vi "V7310.Main-Start.vi"(8 "error in":errorcluster, 9 "Wait (T)":bool=TRUE, 10 "Job":T1) -> (0 "error out":errorcluster, 2 "Aborted":bool)   [LabVIEW 2015]
uses:
  LowLevel/V7310.Job.Data.ctl
  LowLevel/V7310.Job.Sets.ctl
  tools/EventLog/EventLog.EventSource.ctl
  tools/Translator/Translator.Message.ctl
  V7310.Action.ctl
  V7310.Data.Status.State.ctl
  LowLevel/V7310.LaserStatus.ctl
  tools/EventLog/EventLog.CreateError(array).vi
  tools/Translator/Translator.Translate.Status (NoError).vi
  tools/Translator/Translator.FormatMessage.vi
  LowLevel/V7310.Global.vi
  tools/Translator/Translator.Global.vi
  tools/ErrorHandling/ErrorHandling.Create.vi
  tools/EventLog/EventLog.CreateError(single).vi
panel:
  out "delays":u32[](array[numeric])
  out "idx":i32
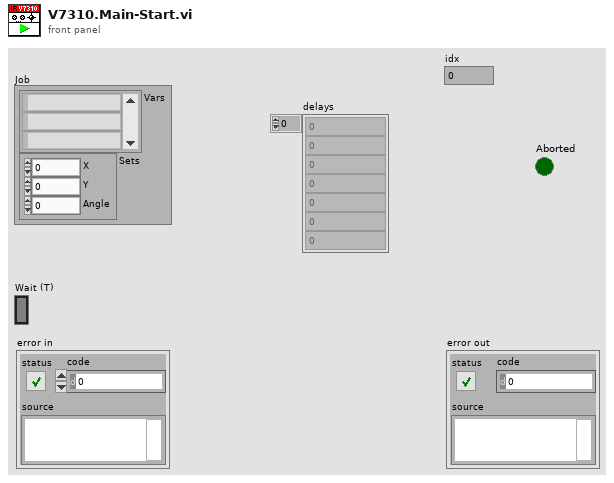
[diagram p1: front panel]
types:
  T1 = typedef "V7310.Job.Data.ctl" = cluster{"Vars":string[], "Sets":T2}
  T2 = typedef "V7310.Job.Sets.ctl" = cluster{"X":dbl, "Y":dbl, "Angle":dbl}
  T3 = typedef "EventLog.EventSource.ctl" = enum16{"All", "Gui", "Ref", "File", "Arch", "Seq", "CPX", "Proda", "Laser", "Scan.P", "Scan.O"}
  T4 = typedef "Translator.Message.ctl" = enum16{"-", "Event confirmed", "Log out", "Log in", "Shutdown", "Cancel", "Start", "Begin time", "End time", "Duration", "Service Mode", "Ignore Results", "On", "Off", "OK", "NOK", "NOK %s", "Home", "Work", "Close", "Open", "In progress...", "Missing", "Empty", "Hardware failure", "Initial", "Out of range", "Error %d >> %s", "Error %d >> %s >> %s", "Msg %d >> %s", "Laser msg %d %s", "Laser cmd error %s %d", "Laser cmd failed %s", "Laser cmd warning %s", "Laser disconnected", "Laser status %s", "Laser already started", "Laser job unkonwn %s", "Laser job missing %s", "Laser job select failure %s", "Unable to start laser printing (%s)", "Unable to stop laser printing (%s)", "Laser marking aborted", "Laser marking timeout", "Unable to reset Laser Interlock (%s)", "Unable to trigger Laser. Laser not ready (%s)", "Laser job '%s' coordinates not configured", "Starting %s", "Quitting %s", "Configured", "Initializing", "Quitting", "Loading", "Running", "Stopped", "Summary", "Laser", "Do you want to continue?", "Press confirm button", "Station is not based. Do you want to exit?", "Station requires changeover. Do you want to run the test?", "Test options are not set as default. Do you want to continue?", "Product not detected. Do you want to continue?", "Product scan failed. Do you want to continue?", "Calibration", "Log out?", "System", "All", "IDLE", "Translating...%s", "Not found", "Alarm %s", "Run", "Skip", "Abort", "Repeat", "Please wait...", "Database disconnected", "Database disconnected - changeover disabled!", "Login to database successful", "Login to database failed: %d; %s", "Unable to check the product status of reference %d - database disconnected", "Unable to set the product status of reference %d - database disconnected", "Variant file backup %s", "Read steps (%s)", "Result", "Station armed!", "Station requires changeover!", "Select reference number...", "EMERGENCY BUTTON - press Control button", "EMERGENCY DOOR - press Control button", "Resetting Emergency...", "Unable to reset safety circuit - Emergency Button pressed", "Unable to reset safety circuit - Emergency Side Door open", "Station not based", "Station based", "Station not empty", "Station basing...", "No order", "Press Start to begin new order", "Scanning new order", "Order NOK. Correct or scan again", "Order OK. Press Accept", "Order ready", "Revolver incorrect", "Fork incorrect", "Revolver missing", "Revolver empty", "Container missing", "Offline results", "Door open", "Close the front door", "Press start button", "Done. Open the front door", "Running...", "Running...%.1f %%", "Pause", "Pause. NOK container missing", "Pause. OK container missing", "Pause. Revolver empty", "Pause. Revolver missing", "Pause. Revolver incorrect", "Pause. Fork missing", "Pause. Fork incorrect", "Pause. Too many failures", "Pause. One slot is not working", "Pause. Unable to move product to slot", "Pause. Unable to move back product pusher", "Pause. Unable to lift product", "Pause. Unable to move back product lifter", "Pause. Unable to move product arm to Work", "Pause. Unable to move product arm to NOK", "Pause. Unable to move product arm to OK", "Pause. Unable to unsuck the NOK product", "Pause. Unable to drop the NOK product", "Pause. Product OK missing", "Pause. Unable to unsuck the OK product", "Pause. Unable to drop the OK product", "Stopping...", "File '%s' is missing", "File '%s' is broken", "File '%s' is running", "Log file started (%s)", "Log file ended (%s)", "Log file ignored (%s)", "Log file exported (%s)", "Log file export failed (%s)", "Wrong serial number in log file", "Wrong reference number in log file", "Test steps are missing", "%s = %.3f", "Process param '%s' not found in DB", "Process param '%s' wrong order", "Process param '%s' value %.3f out of limits (%.3f; %.3f)", "Step%d param '%s' not found in DB", "Step%d param '%s' wrong order", "Step%d param '%s' value %.3f out of limits (%.3f; %.3f)", "Step%d EV '%s' not found in DB", "Step%d EV '%s' wrong order", "\"%s\" not found in DB", "\"%s\" wrong order", "\"%s\" value %.3f out of limits (%.3f; %.3f)", "\"%s\" not found in software", "Process init (%s)", "Process started", "Process restarted", "Process run", "Process done", "Process aborted", "Process aborted at work", "Process aborted at home", "Process error", "Process error at home", "Process error at work", "Process close", "Select plate from the order to process", "Do you want to start the process?", "Do you want to repeat the process?", "There is unfinished order. Do you want to put the new order?", "Product %s %d OK", "Product %s %d NOK", "Unable to unload the slot %s. Product missing in the slot", "Unable to unload the slot %s. Product already in the arm", "Unable to accept the product as OK. Product missing in slot %s", "Unable to accept the product as OK. Product could not drop into the container at slot %s", "Unable to accept the product as NOK. Product could not drop into the container at slot %s", "Scan failed. Error %s", "Scan failed. Scanner disconnected", "Scan failed. Wrong Wabco number %d, limit (%d,%d)", "Scan failed. Wrong serial number %d, limit (%d,%d)", "Scan failed. Wrong date %d, limit (%d,%d)", "Scan failed. Wrong product wabco number %d (expected %d)", "Scan failed. Wrong product serial number %d (expected > 0)", "Scan OK %s", "Scan failed. Unable to determine table position (%s)", "Scan failed. Timeout", "Tune failed. Scanner disconnected", "Tune failed. Timeout", "%s = %d", "%s = %d->%d", "Unable to set %s = %.2f - Air Pressure Inside off", "Unable to set digital output '%s' = %d", "Unable to activate air pressure inside - timeout", "Unable to activate air pressure inside - aborted", "Unable to switch on Air Main Valve - Air Pressure Inlet off", "Unable to switch on Air Main Valve - Door open", "Unable to switch off Air Main Valve - timeout", "Unable to switch off Air Main Valve - aborted", "Unable to rotate Table - timeout", "Unable to rotate Table - aborted", "Unable to rotate Table - Product Move not in Home position", "Unable to rotate Table - Air Pressure Inside off", "Unable to rotate Table - Product Lift A not in Home position", "Unable to rotate Table - Product Lift B not in Home position", "Unable to rotate Table - unlock before movement timeout", "Unable to rotate Table - lock after movement timeout", "Unable to move Table Lock to %s position - timeout", "Unable to move Table Lock to %s position - aborted", "Unable to move Table Lock to %s position - Air Pressure Inside off", "Unable to move Table Lock to %s position - Table not in position", "Unable to move Product Lift A to %s position - timeout", "Unable to move Product Lift B to %s position - timeout", "Unable to move Product Lift A to %s position - aborted", "Unable to move Product Lift B to %s position - aborted", "Unable to move Product Lift A to %s position - Air Pressure Inside off", "Unable to move Product Lift B to %s position - Air Pressure Inside off", "Unable to move Product Lift A to %s position - Table not locked", "Unable to move Product Lift B to %s position - Table not locked", "Unable to move Product Lift A to %s position - Product Arm not in Work position", "Unable to move Product Lift B to %s position - Product Arm not in Work position", "Unable to set Product Suction Gripper %s to %s - timeout", "Unable to set Product Suction Gripper %s to %s - aborted", "Unable to set Product Suction Gripper %s to %s - Air Pressure Inside off", "Unable to set Product Suction Gripper %s to %s - Table slot unkown", "Unable to move Product Arm to %s position - timeout", "Unable to move Product Arm to %s position - aborted", "Unable to move Product Arm to %s position - Air Pressure Inside off", "Unable to move Product Arm to %s position - Product Lift A not in Home position", "Unable to move Product Arm to %s position - Product Lift B not in Home position", "Unable to move Product to %s position - timeout", "Unable to move Product to %s position - aborted", "Unable to move Product to %s position - Air Pressure Inside off", "Unable to move Product to %s position - Table not in position"}
  T5 = typedef "V7310.Action.ctl" = enum32{"idle", "constructor", "destructor", "--- V7310 ---", "Init", "Select", "Start", "Stop"}
  T6 = typedef "V7310.Data.Status.State.ctl" = enum16{"First", "Init", "Msg", "Error", "Abort", "Idle", "Run"}
  T7 = typedef "V7310.LaserStatus.ctl" = enum16{"-", "FatalError", "Initialize", "KeySwitchOpen", "TimeoutInterlock", "InterlockOpen", "StartUp", "ShutterlockOpen", "Standby", "Ready", "PrepareForMarking", "WaitForTrigger", "Marking"}
  T8 = typedef "V7310.Data.Status.ctl" = cluster{"State":T6, "LaserStatus":T7, "LaserStatusRaw":string, "Ref":refnum<k5>, "RTC TS":timestamp, "Conn TS":timestamp, "Msg":T9[], "JobInUse":string, "Jobs":string[], "Vars":T10[]}
  T9 = typedef "V7310.Message.Data.ctl" = cluster{"ID":i32, "Msg":string}
  T10 = typedef "V7310.Job.Variable.ctl" = cluster{"Name":string, "Value":string}
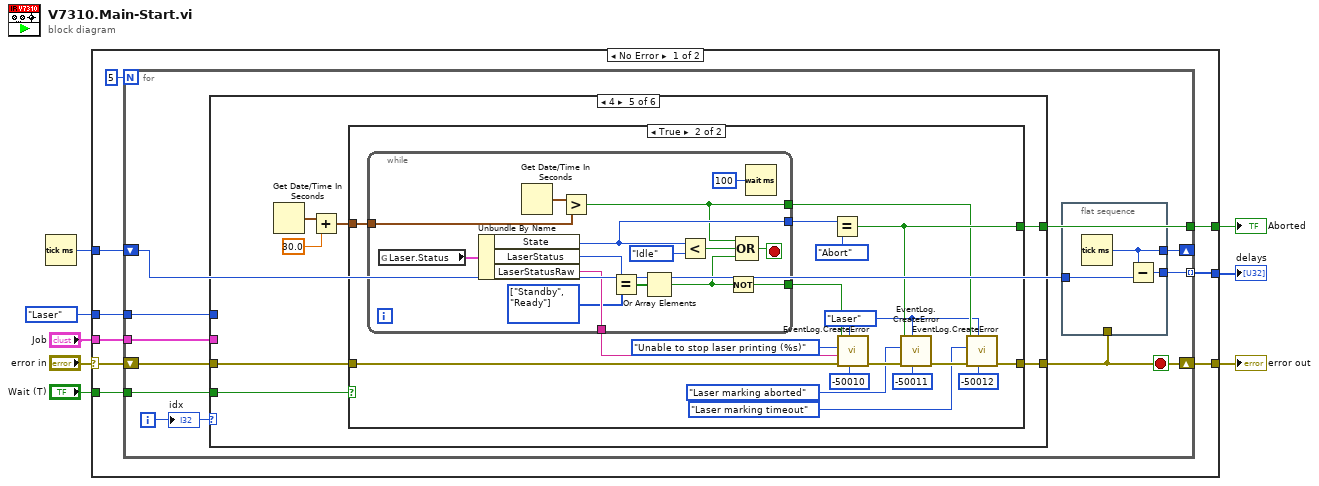
[diagram p0: block diagram]
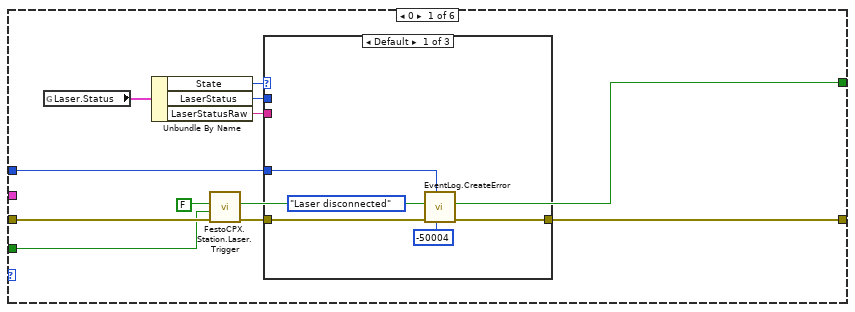
[diagram p2: hidden frame]
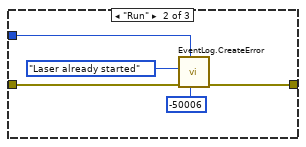
[diagram p3: hidden frame]
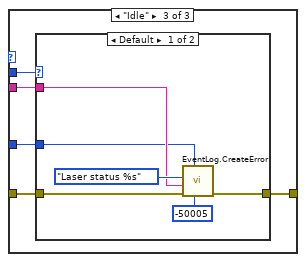
[diagram p4: hidden frame]
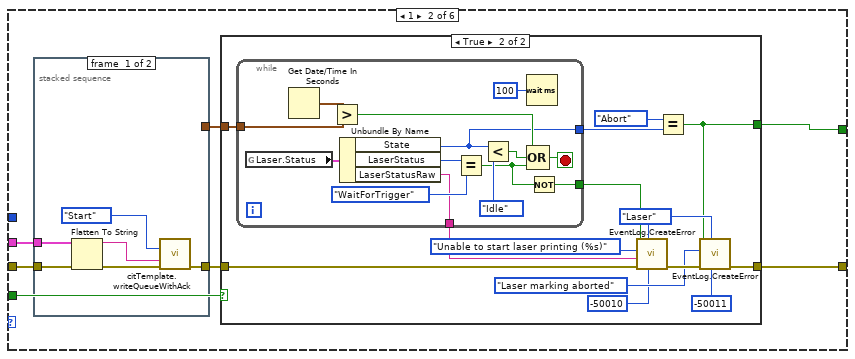
[diagram p6: hidden frame]
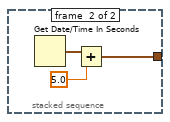
[diagram p7: hidden frame]
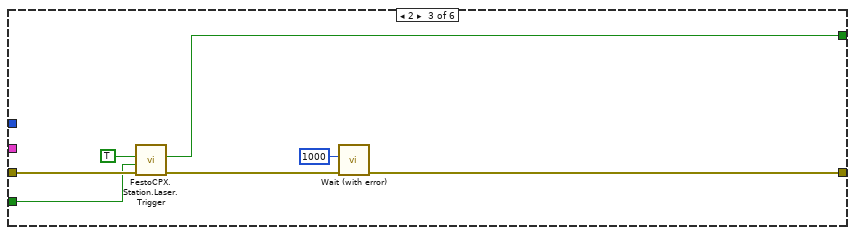
[diagram p9: hidden frame]
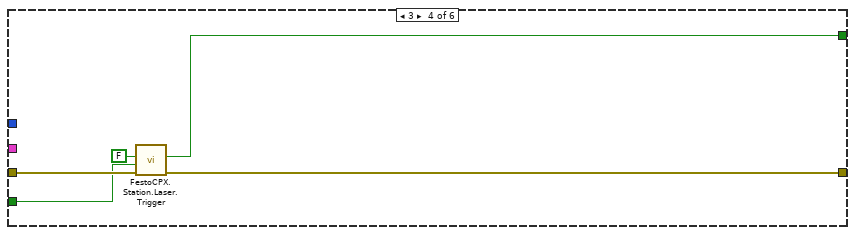
[diagram p10: hidden frame]
diagram:
  n1 = Tick Count (ms)() -> (millisecond timer value=w2:u32)
  n2 = case shown="No Error" "error in" {
    selector: "error in" -> [w15 w163]
    tunnel: [w16 w163] -> w7
    tunnel: "Job" -> [w17 _]
    tunnel: "Wait (T)" -> [w14 _]
    tunnel: [w11 _] -> w4
    tunnel: EventLog.EventSource."Laser" ("Source (All)") -> [w13 _]
    tunnel: w2 -> [w10 _]
    tunnel: [w9 _] -> w1
    frame No Error {
      n3 = for {
        N: 5 -> [_]
        tunnel: w17 -> [w27]
        shift-right: [w21] -> w16
        shift-left: w15 -> [w26]
        tunnel: w14 -> [w25]
        tunnel: w13 -> [w23]
        tunnel: [w22] -> w11
        shift-right: [w20] -> _
        shift-left: w10 -> [w19]
        tunnel: [w18] -> w9 mode=indexing
        i -> [w24]
        stop <- w21 stop-if-true
        n4 = case shown="4" w24 {
          tunnel: w27 -> [_ w70 _ _ _ _]
          tunnel: [w41 w65 w110 w118 w125 w162] -> w21
          tunnel: w26 -> [w37 w69 w114 w119 w121 w162]
          tunnel: w25 -> [w32 w68 w112 w117 w127 _]
          tunnel: w23 -> [w34 _ _ _ _ _]
          tunnel: [w31 w64 w111 w116 w124 _] -> w22
          frame 0 {
            n5 = global read "V7310.Global.vi" "Laser.Status"() -> (w33:T8)
            n6 = Unbundle By Name(w33) -> ("State"=w40:T6, "LaserStatus"=w39:T7, "LaserStatusRaw"=w38:string)
            n7 = call "FestoCPX.Station.Laser.Trigger.vi"("error in"=w37, "Wait (T)"=w32, "Trigger"=FALSE) -> ("error out"=w36:errorcluster, "Aborted"=w31:bool)  [unwired: 7 in]
            n8 = case shown="Default" w40 {
              tunnel: w36 -> [w44 w50 w56]
              tunnel: [w43 w49 w55] -> w41
              tunnel: w39 -> [_ _ w54]
              tunnel: w38 -> [_ _ w53]
              tunnel: w34 -> [w42 w47 w52]
              frame Default {
                n9 = call-poly "EventLog.CreateError.vi"("Code (-1)"=-50004 ("error code (0)"), "Source (All)"=w42, "error in"=w44, "msg"=Translator.Message."Laser disconnected") -> ("error out"=w43:errorcluster)  [unwired: 6 in, 1 out]
              }
              frame "Run" {
                n10 = call-poly "EventLog.CreateError.vi"("Code (-1)"=-50006 ("error code (0)"), "Source (All)"=w47, "error in"=w50, "msg"=Translator.Message."Laser already started") -> ("error out"=w49:errorcluster)  [unwired: 6 in, 1 out]
              }
              frame "Idle" {
                n11 = case shown="Default" w54 {
                  tunnel: w56 -> [w60 w63]
                  tunnel: [w59 w63] -> w55
                  tunnel: w53 -> [w58 _]
                  tunnel: w52 -> [w57 _]
                  frame Default {
                    n12 = call-poly "EventLog.CreateError.vi"("Code (-1)"=-50005 ("error code (0)"), "Source (All)"=w57, "error in"=w60, "arg"=w58, "msg"=Translator.Message."Laser status %s") -> ("error out"=w59:errorcluster)  [unwired: 6 in]
                  }
                  frame "Standby", "Ready" {
                  }
                }
              }
            }
          }
          frame 1 {
            n13 = stacked-sequence {
              tunnel: w69 -> [w76 _]
              tunnel: w70 -> [w73 _]
              tunnel: [w71 _] -> w67
              tunnel: [_ w77] -> w66
              frame #0 {
                n14 = Flatten To String(anything=w73, error in (no error)=w76) -> (data string=w74:string, error out=w75:errorcluster)  [unwired: 2 in, 1 out]
                n15 = call "citTemplate.writeQueueWithAck.vi"("event in"=V7310.Action."Start" ("Action"), "(flatten) data in"=w74, "error in (no error)"=w75) -> ("error out"=w71:errorcluster)  [unwired: 10 in, 2 out]
              }
              frame #1 {
                n16 = Get Date/Time In Seconds() -> (seconds since 1Jan1904=w79:timestamp)
                n17 = Add(x=w79, y=5.0 ("x")) -> (x+y=w77:timestamp)
              }
            }
            n18 = case shown="True" w68 {
              tunnel: w67 -> [w80 w92]
              tunnel: [w80 w89] -> w65
              tunnel: w66 -> [_ w94]
              tunnel: [_ w85] -> w64
              frame False {
              }
              frame True {
                w87 = EventLog.EventSource."Laser" ("Source (All)")
                n19 = while {
                  tunnel: w94 -> [w103]
                  tunnel: [w98] -> w93
                  tunnel: [w96] -> w91
                  tunnel: [w95] -> w81
                  stop <- w100 stop-if-true
                  n20 = global read "V7310.Global.vi" "Laser.Status"() -> (w108:T8)
                  n21 = Get Date/Time In Seconds() -> (seconds since 1Jan1904=w102:timestamp)
                  n22 = Greater?(x=w102, y=w103) -> (0:w101:bool)
                  n23 = Unbundle By Name(w108) -> ("State"=w96:T6, "LaserStatus"=w107:T7, "LaserStatusRaw"=w95:string)
                  n24 = Equal?(x=w107, y=V7310.LaserStatus."WaitForTrigger") -> (x = y?=w99:bool)
                  n25 = Less?(x=w96, y=V7310.Data.Status.State."Idle" ("State")) -> (x < y?=w104:bool)
                  n26 = Wait (ms)(milliseconds to wait=u32 100) -> ()  [unwired: 1 out]
                  n27 = Compound Arithmetic op=OR(w101, w104, w99) -> (w100:bool)
                  n28 = Not(x=w99) -> (.not. x?=w98:bool)
                }
                n29 = call-poly "EventLog.CreateError.vi"("Code (-1)"=-50010, "Source (All)"=w87, "error in"=w92, "arg"=w81, "msg"=Translator.Message."Unable to start laser printing (%s)", "create (T)"=w93) -> ("error out"=w88:errorcluster)  [unwired: 5 in]
                n30 = Equal?(x=V7310.Data.Status.State."Abort", y=w91) -> (x = y?=w85:bool)
                n31 = call-poly "EventLog.CreateError.vi"("Code (-1)"=-50011, "Source (All)"=w87, "error in"=w88, "msg"=Translator.Message."Laser marking aborted", "create (T)"=w85) -> ("error out"=w89:errorcluster)  [unwired: 5 in, 1 out]
              }
            }
          }
          frame 2 {
            n32 = call "FestoCPX.Station.Laser.Trigger.vi"("error in"=w114, "Wait (T)"=w112, "Trigger"=TRUE) -> ("error out"=w113:errorcluster, "Aborted"=w111:bool)  [unwired: 7 in]
            n33 = call "Wait (with error).vi"("error in (no error)"=w113, "milliseconds to wait"=u32 1000) -> ("error out"=w110:errorcluster)  [unwired: 8 in, 1 out]
          }
          frame 3 {
            n34 = call "FestoCPX.Station.Laser.Trigger.vi"("error in"=w119, "Wait (T)"=w117, "Trigger"=FALSE) -> ("error out"=w118:errorcluster, "Aborted"=w116:bool)  [unwired: 7 in]
          }
          frame 4 {
            n35 = Get Date/Time In Seconds() -> (seconds since 1Jan1904=w123:timestamp)
            n36 = Add(x=w123, y=30.0 ("x")) -> (x+y=w126:timestamp)
            n37 = case shown="True" w127 {
              tunnel: w121 -> [w128 w144]
              tunnel: [w128 w132] -> w125
              tunnel: w126 -> [_ w146]
              tunnel: [_ w138] -> w124
              frame False {
              }
              frame True {
                w130 = EventLog.EventSource."Laser" ("Source (All)")
                n38 = while {
                  tunnel: w146 -> [w158]
                  tunnel: [w151] -> w145
                  tunnel: [w154] -> w142
                  tunnel: [w149] -> w135
                  tunnel: [w147] -> w131
                  stop <- w156 stop-if-true
                  w148 = T7[] [enum."Standby", enum."Ready"] items=["-", "FatalError", "Initialize", "KeySwitchOpen", "TimeoutInterlock", "InterlockOpen", "StartUp", "ShutterlockOpen", "Standby", "Ready", "PrepareForMarking", "WaitForTrigger", "Marking"]
                  n39 = global read "V7310.Global.vi" "Laser.Status"() -> (w161:T8)
                  n40 = Unbundle By Name(w161) -> ("State"=w154:T6, "LaserStatus"=w152:T7, "LaserStatusRaw"=w149:string)
                  n41 = Get Date/Time In Seconds() -> (seconds since 1Jan1904=w157:timestamp)
                  n42 = Greater?(x=w157, y=w158) -> (0:w147:bool)
                  n43 = Equal?(x=w152, y=w148) -> (x = y?=w153:bool[])
                  n44 = Or Array Elements(Boolean array=w153) -> (logical OR=w150:bool)
                  n45 = Less?(x=w154, y=V7310.Data.Status.State."Idle" ("State")) -> (x < y?=w159:bool)
                  n46 = Not(x=w150) -> (.not. x?=w151:bool)
                  n47 = Compound Arithmetic op=OR(w147, w159, w150) -> (w156:bool)
                  n48 = Wait (ms)(milliseconds to wait=u32 100) -> ()  [unwired: 1 out]
                }
                n49 = Equal?(x=w142, y=V7310.Data.Status.State."Abort" ("x")) -> (x = y?=w138:bool)
                n50 = call-poly "EventLog.CreateError.vi"("Code (-1)"=-50010, "Source (All)"=w130, "error in"=w144, "arg"=w135, "msg"=Translator.Message."Unable to stop laser printing (%s)", "create (T)"=w145) -> ("error out"=w140:errorcluster)  [unwired: 5 in]
                n51 = call-poly "EventLog.CreateError.vi"("Code (-1)"=-50011, "Source (All)"=w130, "error in"=w140, "msg"=Translator.Message."Laser marking aborted", "create (T)"=w138) -> ("error out"=w133:errorcluster)  [unwired: 5 in, 1 out]
                n52 = call-poly "EventLog.CreateError.vi"("Code (-1)"=-50012, "Source (All)"=w130, "error in"=w133, "msg"=Translator.Message."Laser marking timeout", "create (T)"=w131) -> ("error out"=w132:errorcluster)  [unwired: 5 in, 1 out]
              }
            }
          }
          frame Default {
          }
        }
        n53 = flat-sequence {
          tunnel: w21 -> [_]
          tunnel: w19 -> [w30]
          tunnel: [w29] -> w20
          tunnel: [w28] -> w18
          frame #0 {
            n54 = Tick Count (ms)() -> (millisecond timer value=w29:u32)
            n55 = Subtract(x=w29, y=w30) -> (x-y=w28:u32)
          }
        }
        "idx" <- w24
      }
    }
    frame Error {
    }
  }
  "error out" <- w7
  "Aborted" <- w4
  "delays" <- w1
